vi "TestArena.vi"() -> ()   [LabVIEW 2013]
panel:
  out "Distance Chart 2":dbl(graph)
  in  "stop":bool
  in  "Speed (mm/s)":dbl
  out "Output 1 Chart":dbl(graph)
  out "Speed Output (mm/s) 1":dbl
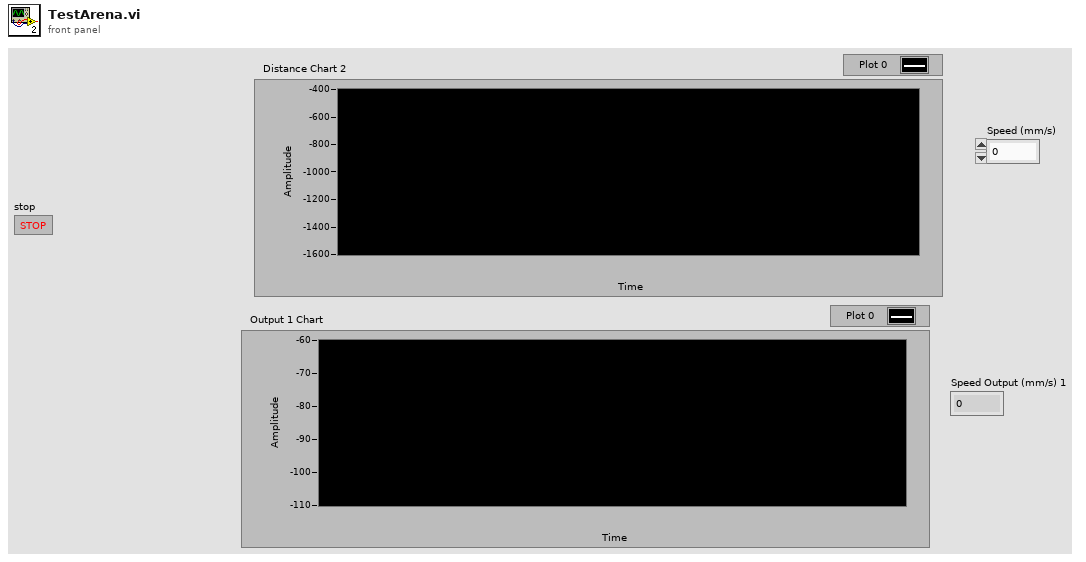
[diagram p1: front panel]
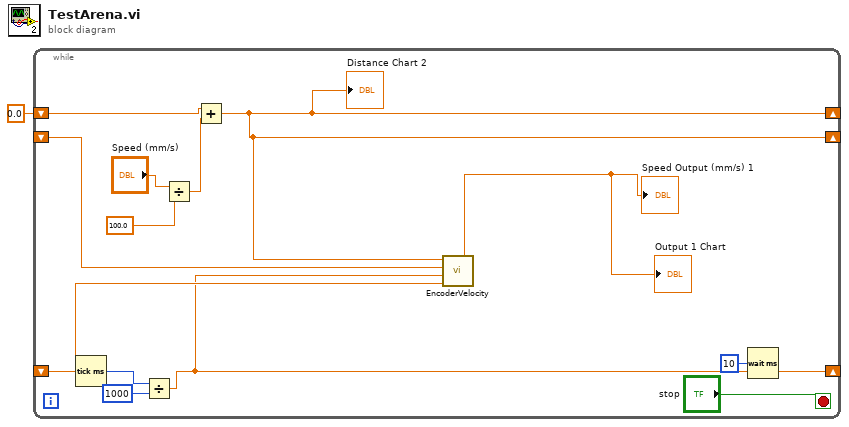
[diagram p0: block diagram]
diagram:
  n1 = while {
    shift-right: [w8] -> _
    shift-left: 0.0 -> [w12]
    shift-right: [w8] -> _
    shift-left: _ -> [w11]
    shift-right: [w6] -> _
    shift-left: _ -> [w10]
    stop <- "stop" stop-if-true
    n2 = Tick Count (ms)() -> (millisecond timer value=w7:u32)
    n3 = Divide(x=w7, y=u32 1000) -> (x/y=w6:dbl)
    n4 = Divide(x="Speed (mm/s)", y=100.0) -> (x/y=w3:dbl)
    n5 = Add(x=w12, y=w3) -> (x+y=w8:dbl)
    "Distance Chart 2" <- w8
    n6 = call "EncoderVelocity.vi"("Time @(n-1)"=w10, "Time @n"=w6, "Encoder Distance (mm) @n-1"=w11, "Encoder Distance (mm) @n"=w8) -> ("Encoder Speed (mm/s)"=→"Speed Output (mm/s) 1" →"Output 1 Chart":dbl)  [unwired: 7 in]
    n7 = Wait (ms)(milliseconds to wait=u32 10) -> ()  [unwired: 1 out]
  }
